vi "testTimer.vi"(8 "error in (no error)":errorcluster) -> (0 "error out":errorcluster, 4 "relative seconds":dbl)   [LabVIEW 2020]
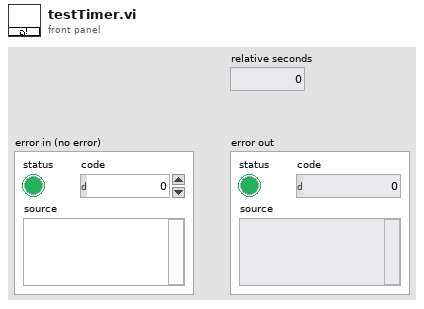
[diagram p1: front panel]
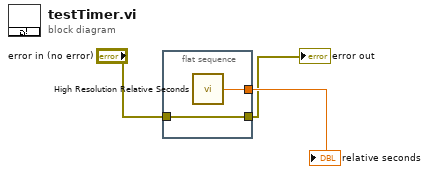
[diagram p0: block diagram]
diagram:
  n1 = flat-sequence {
    tunnel: "error in (no error)" -> [w5]
    tunnel: [w5] -> w2
    tunnel: [w4] -> w3
    frame #0 {
      n2 = call <vilib>:"High Resolution Relative Seconds.vi"() -> ("relative seconds"=w4:dbl)
    }
  }
  "relative seconds" <- w3
  "error out" <- w2
